vi "Delay.vi"(7 "Delay":u32=500, 8 "error in (no error)":errorcluster) -> (0 "error out":errorcluster)   [LabVIEW 2018]
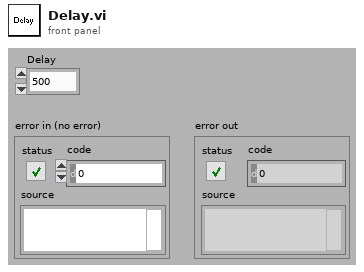
[diagram p1: front panel]
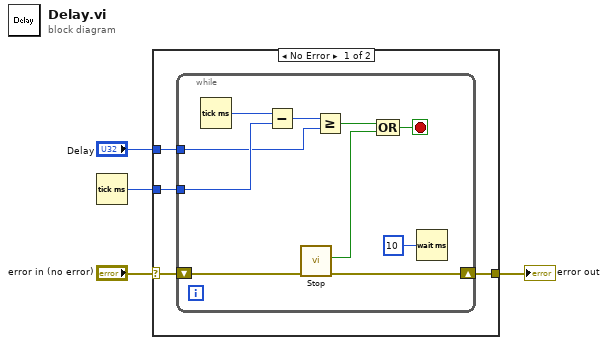
[diagram p0: block diagram]
diagram:
  n1 = Tick Count (ms)() -> (millisecond timer value=w4:u32)
  n2 = case shown="No Error" "error in (no error)" {
    selector: "error in (no error)" -> [w5 w19]
    tunnel: w4 -> [w8 _]
    tunnel: "Delay" -> [w7 _]
    tunnel: [w6 w19] -> w2
    frame No Error {
      n3 = while {
        tunnel: w8 -> [w17]
        tunnel: w7 -> [w15]
        shift-right: [w9] -> w6
        shift-left: w5 -> [w13]
        stop <- w11 stop-if-true
        n4 = Tick Count (ms)() -> (millisecond timer value=w18:u32)
        n5 = Subtract(x=w18, y=w17) -> (x-y=w16:u32)
        n6 = call "Stop.vi"("error in (no error)"=w13) -> ("error out"=w9:errorcluster, "StateOut"=w10:bool)  [unwired: 9 in]
        n7 = Greater Or Equal?(x=w16, y=w15) -> (x >= y?=w12:bool)
        n8 = Compound Arithmetic op=OR(w12, w10) -> (w11:bool)
        n9 = Wait (ms)(milliseconds to wait=u32 10) -> ()  [unwired: 1 out]
      }
    }
    frame Error {
    }
  }
  "error out" <- w2
